vi "Read Local IP Address.vi"(8 "error in (no error)":errorcluster, 11 "UDP in":refnum<class "UDP.lvclass">) -> (0 "error out":errorcluster, 2 "Local IP Address":string, 3 "UDP out":refnum<class "UDP.lvclass">)   [LabVIEW 2013, in "Protocol Classes.lvlib" / "UDP.lvclass"]
uses:
  UDP.lvclass
  UDP.lvclass/UDP.ctl
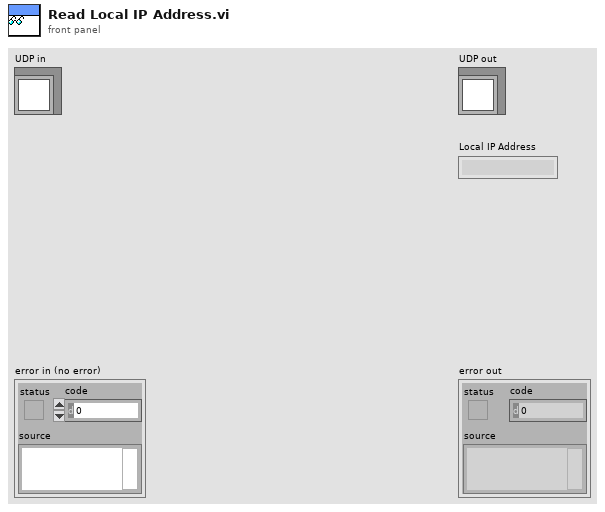
[diagram p1: front panel]
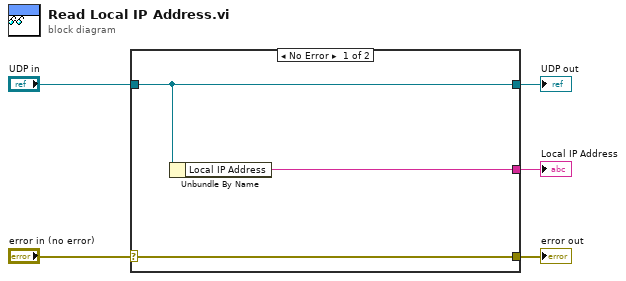
[diagram p0: block diagram]
diagram:
  n1 = case shown="No Error" "error in (no error)" {
    selector: "error in (no error)" -> [w8 w9]
    tunnel: [w8 w9] -> w4
    tunnel: [w7 w10] -> w2
    tunnel: "UDP in" -> [w7 w10]
    tunnel: [w6 _] -> w1
    frame No Error {
      n2 = Unbundle By Name(w7) -> ("Local IP Address"=w6:string)
    }
    frame Error {
    }
  }
  "error out" <- w4
  "UDP out" <- w2
  "Local IP Address" <- w1
